vi "Photo_Editor_Project_EE304.vi"() -> ()   [LabVIEW 2019]
panel:
  in  "Save Button":bool
  in  "Blue":i32(slide) scale=0.0..100.0
  in  "Green":i32(slide) scale=0.0..100.0
  in  "Red":i32(slide) scale=0.0..100.0
  in  "Zoom to Fit Canvas":sgl
  out "Image":picture
  in  "Balance Button":bool
  in  "Shadows":i32(slide) scale=0.0..10.0
  in  "Highlights":i32(slide) scale=0.0..10.0
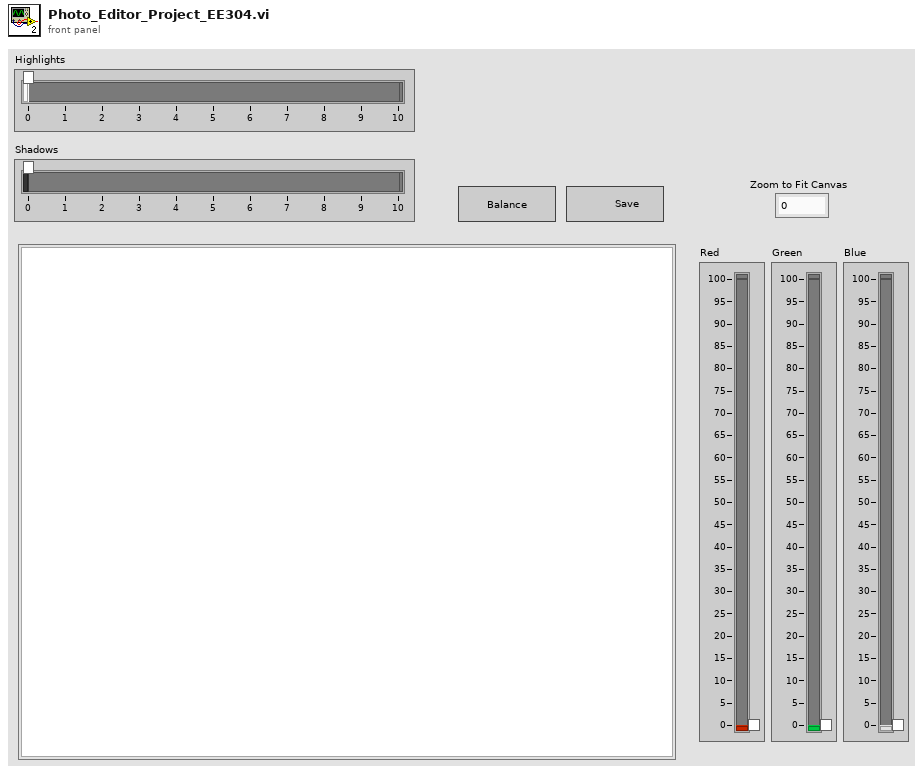
[diagram p1: front panel]
types:
  T1 = typedef "imagedata.ctl" = cluster{"image type":i32, "image depth":i32, "image":u8[], "mask":u8[], "colors":u32[], "Rectangle":cluster{"left":i16, "top":i16, "right":i16, "bottom":i16}}
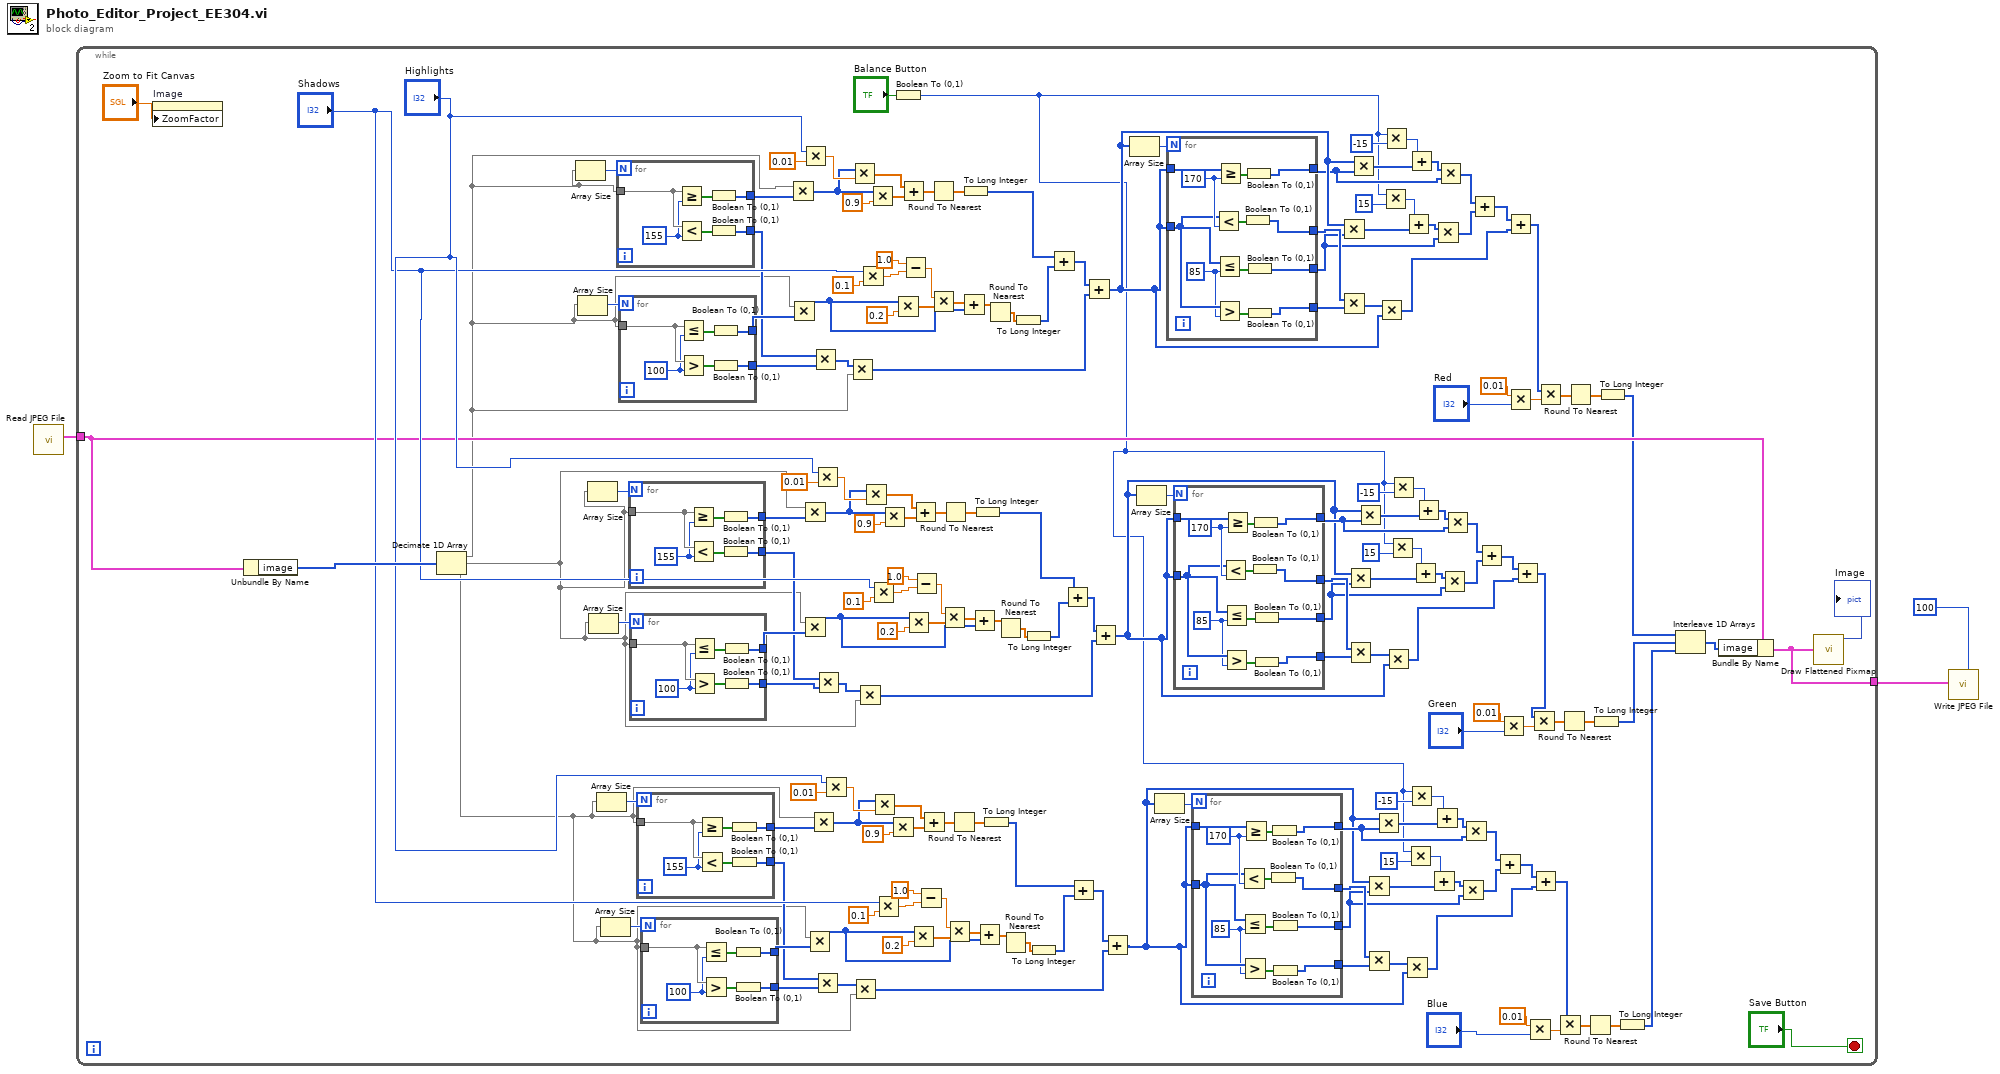
[diagram p0: block diagram]
diagram:
  n1 = call <vilib>:"Read JPEG File.vi"() -> ("image data"=w3:T1)  [unwired: 9 in, 2 out]
  n2 = while {
    tunnel: w3 -> [w90]
    tunnel: [w5] -> w1
    stop <- "Save Button" stop-if-true
    n3 = property on="Image" class="Pict"("ZoomFactor"="Zoom to Fit Canvas") -> ()  [unwired: 2 in, 2 out]
    n4 = Unbundle By Name(w90) -> ("image"=w182:u8[])
    n5 = Decimate 1D Array(w182) -> (w70:u8[], w50:u8[], w29:u8[])
    n6 = Array Size(array=w70) -> (size(s)=w169:i32)
    n7 = Array Size(array=w70) -> (size(s)=w148:i32)
    n8 = Array Size(array=w50) -> (size(s)=w180:i32)
    n9 = Array Size(array=w50) -> (size(s)=w135:i32)
    n10 = Array Size(array=w29) -> (size(s)=w158:i32)
    n11 = Array Size(array=w29) -> (size(s)=w123:i32)
    n12 = for {
      N: w169 -> [_]
      tunnel: w70 -> [w246]
      tunnel: [w247] -> w168
      tunnel: [w243] -> w109
      w245 = u8 155 ("y")
      n13 = Greater Or Equal?(x=w246, y=w245) -> (x >= y?=w248:bool[])
      n14 = Less?(x=w246, y=w245) -> (x < y?=w244:bool[])
      n15 = Boolean To (0,1)(Boolean=w248) -> (0, 1=w247:i16[])
      n16 = Boolean To (0,1)(Boolean=w244) -> (0, 1=w243:i16[])
    }
    n17 = for {
      N: w148 -> [_]
      tunnel: w70 -> [w234]
      tunnel: [w235] -> w146
      tunnel: [w231] -> w108
      w233 = u8 100 ("y")
      n18 = Less Or Equal?(x=w234, y=w233) -> (x <= y?=w236:bool[])
      n19 = Greater?(x=w234, y=w233) -> (0:w232:bool[])
      n20 = Boolean To (0,1)(Boolean=w236) -> (0, 1=w235:i16[])
      n21 = Boolean To (0,1)(Boolean=w232) -> (0, 1=w231:i16[])
    }
    n22 = for {
      N: w180 -> [_]
      tunnel: w50 -> [w252]
      tunnel: [w253] -> w179
      tunnel: [w249] -> w102
      w251 = u8 155 ("y")
      n23 = Greater Or Equal?(x=w252, y=w251) -> (x >= y?=w254:bool[])
      n24 = Less?(x=w252, y=w251) -> (x < y?=w250:bool[])
      n25 = Boolean To (0,1)(Boolean=w254) -> (0, 1=w253:i16[])
      n26 = Boolean To (0,1)(Boolean=w250) -> (0, 1=w249:i16[])
    }
    n27 = for {
      N: w135 -> [_]
      tunnel: w50 -> [w228]
      tunnel: [w229] -> w134
      tunnel: [w225] -> w103
      w227 = u8 100 ("y")
      n28 = Less Or Equal?(x=w228, y=w227) -> (x <= y?=w230:bool[])
      n29 = Greater?(x=w228, y=w227) -> (0:w226:bool[])
      n30 = Boolean To (0,1)(Boolean=w230) -> (0, 1=w229:i16[])
      n31 = Boolean To (0,1)(Boolean=w226) -> (0, 1=w225:i16[])
    }
    n32 = for {
      N: w158 -> [_]
      tunnel: w29 -> [w240]
      tunnel: [w241] -> w157
      tunnel: [w237] -> w98
      w239 = u8 155 ("y")
      n33 = Greater Or Equal?(x=w240, y=w239) -> (x >= y?=w242:bool[])
      n34 = Less?(x=w240, y=w239) -> (x < y?=w238:bool[])
      n35 = Boolean To (0,1)(Boolean=w242) -> (0, 1=w241:i16[])
      n36 = Boolean To (0,1)(Boolean=w238) -> (0, 1=w237:i16[])
    }
    n37 = for {
      N: w123 -> [_]
      tunnel: w29 -> [w222]
      tunnel: [w223] -> w122
      tunnel: [w219] -> w97
      w221 = u8 100 ("y")
      n38 = Less Or Equal?(x=w222, y=w221) -> (x <= y?=w224:bool[])
      n39 = Greater?(x=w222, y=w221) -> (0:w220:bool[])
      n40 = Boolean To (0,1)(Boolean=w224) -> (0, 1=w223:i16[])
      n41 = Boolean To (0,1)(Boolean=w220) -> (0, 1=w219:i16[])
    }
    n42 = Multiply(x=w70, y=w168) -> (x*y=w163:i16[])
    n43 = Multiply(x=w70, y=w146) -> (x*y=w138:i16[])
    n44 = Multiply(x=w50, y=w179) -> (x*y=w174:i16[])
    n45 = Multiply(x=w50, y=w134) -> (x*y=w126:i16[])
    n46 = Multiply(x="Highlights", y=0.01) -> (x*y=w165:dbl)
    n47 = Multiply(x=w29, y=w122) -> (x*y=w114:i16[])
    n48 = Multiply(x=w29, y=w157) -> (x*y=w152:i16[])
    n49 = Multiply(x=w109, y=w108) -> (x*y=w107:i16[])
    n50 = Multiply(x="Highlights", y=0.01) -> (x*y=w176:dbl)
    n51 = Multiply(x=w98, y=w97) -> (x*y=w94:i16[])
    n52 = Multiply(x=w102, y=w103) -> (x*y=w101:i16[])
    n53 = Multiply(x="Highlights", y=0.01) -> (x*y=w154:dbl)
    n54 = Multiply(x=w107, y=w70) -> (x*y=w105:i16[])
    n55 = Multiply(x=w163, y=w165) -> (x*y=w162:dbl[])
    n56 = Multiply(x=w94, y=w29) -> (x*y=w92:i16[])
    n57 = Multiply(x=w101, y=w50) -> (x*y=w99:i16[])
    n58 = Multiply(x="Shadows", y=0.1) -> (x*y=w143:dbl)
    n59 = Multiply(x=w174, y=w176) -> (x*y=w173:dbl[])
    n60 = Multiply(x=w163, y=0.9) -> (x*y=w161:dbl[])
    n61 = Multiply(x="Shadows", y=0.1) -> (x*y=w131:dbl)
    n62 = Multiply(x=w152, y=w154) -> (x*y=w151:dbl[])
    n63 = Multiply(x="Shadows", y=0.1) -> (x*y=w119:dbl)
    n64 = Multiply(x=w174, y=0.9) -> (x*y=w172:dbl[])
    n65 = Multiply(x=w152, y=0.9) -> (x*y=w150:dbl[])
    n66 = Boolean To (0,1)(Boolean="Balance Button") -> (0, 1=w30:i16)
    n67 = Multiply(x=w138, y=0.2) -> (x*y=w140:dbl[])
    n68 = Add(x=w162, y=w161) -> (x+y=w160:dbl[])
    n69 = Subtract(x=1.0, y=w143) -> (x-y=w141:dbl)
    n70 = Multiply(x=w126, y=0.2) -> (x*y=w128:dbl[])
    n71 = Multiply(x=w114, y=0.2) -> (x*y=w116:dbl[])
    n72 = Add(x=w173, y=w172) -> (x+y=w171:dbl[])
    n73 = Subtract(x=1.0, y=w131) -> (x-y=w129:dbl)
    n74 = Subtract(x=1.0, y=w119) -> (x-y=w117:dbl)
    n75 = Add(x=w151, y=w150) -> (x+y=w149:dbl[])
    n76 = Round To Nearest(number=w160) -> (nearest integer value=w167:dbl[])
    n77 = Multiply(x=w141, y=w140) -> (x*y=w139:dbl[])
    n78 = Multiply(x=w129, y=w128) -> (x*y=w127:dbl[])
    n79 = Round To Nearest(number=w171) -> (nearest integer value=w178:dbl[])
    n80 = Multiply(x=w117, y=w116) -> (x*y=w115:dbl[])
    n81 = Round To Nearest(number=w149) -> (nearest integer value=w156:dbl[])
    n82 = Add(x=w139, y=w138) -> (x+y=w137:dbl[])
    n83 = To Long Integer(number=w167) -> (32bit integer=w159:i32[])
    n84 = Add(x=w127, y=w126) -> (x+y=w125:dbl[])
    n85 = To Long Integer(number=w178) -> (32bit integer=w170:i32[])
    n86 = Add(x=w115, y=w114) -> (x+y=w113:dbl[])
    n87 = To Long Integer(number=w156) -> (32bit integer=w95:i32[])
    n88 = Round To Nearest(number=w137) -> (nearest integer value=w136:dbl[])
    n89 = Round To Nearest(number=w125) -> (nearest integer value=w124:dbl[])
    n90 = Round To Nearest(number=w113) -> (nearest integer value=w112:dbl[])
    n91 = To Long Integer(number=w136) -> (32bit integer=w110:i32[])
    n92 = To Long Integer(number=w124) -> (32bit integer=w104:i32[])
    n93 = To Long Integer(number=w112) -> (32bit integer=w96:i32[])
    n94 = Add(x=w159, y=w110) -> (x+y=w106:i32[])
    n95 = Add(x=w170, y=w104) -> (x+y=w100:i32[])
    n96 = Add(x=w95, y=w96) -> (x+y=w93:i32[])
    n97 = Add(x=w106, y=w105) -> (x+y=w85:i32[])
    n98 = Add(x=w100, y=w99) -> (x+y=w51:i32[])
    n99 = Add(x=w93, y=w92) -> (x+y=w31:i32[])
    n100 = Array Size(array=w85) -> (size(s)=w89:i32)
    n101 = Array Size(array=w51) -> (size(s)=w69:i32)
    n102 = Array Size(array=w31) -> (size(s)=w49:i32)
    n103 = for {
      N: w89 -> [_]
      tunnel: w85 -> [w218]
      tunnel: [w216] -> w80
      tunnel: w85 -> [w212]
      tunnel: [w213] -> w88
      tunnel: [w208] -> w75
      tunnel: [w207] -> w87
      w211 = 85 ("y")
      w215 = 170 ("y")
      n104 = Less?(x=w212, y=w215) -> (x < y?=w214:bool[])
      n105 = Less Or Equal?(x=w212, y=w211) -> (x <= y?=w210:bool[])
      n106 = Greater?(x=w212, y=w211) -> (0:w209:bool[])
      n107 = Greater Or Equal?(x=w218, y=w215) -> (x >= y?=w217:bool[])
      n108 = Boolean To (0,1)(Boolean=w214) -> (0, 1=w213:i16[])
      n109 = Boolean To (0,1)(Boolean=w217) -> (0, 1=w216:i16[])
      n110 = Boolean To (0,1)(Boolean=w210) -> (0, 1=w208:i16[])
      n111 = Boolean To (0,1)(Boolean=w209) -> (0, 1=w207:i16[])
    }
    n112 = for {
      N: w69 -> [_]
      tunnel: w51 -> [w206]
      tunnel: [w204] -> w61
      tunnel: w51 -> [w200]
      tunnel: [w201] -> w68
      tunnel: [w196] -> w56
      tunnel: [w195] -> w67
      w199 = 85 ("y")
      w203 = 170 ("y")
      n113 = Less?(x=w200, y=w203) -> (x < y?=w202:bool[])
      n114 = Less Or Equal?(x=w200, y=w199) -> (x <= y?=w198:bool[])
      n115 = Greater?(x=w200, y=w199) -> (0:w197:bool[])
      n116 = Greater Or Equal?(x=w206, y=w203) -> (x >= y?=w205:bool[])
      n117 = Boolean To (0,1)(Boolean=w202) -> (0, 1=w201:i16[])
      n118 = Boolean To (0,1)(Boolean=w205) -> (0, 1=w204:i16[])
      n119 = Boolean To (0,1)(Boolean=w198) -> (0, 1=w196:i16[])
      n120 = Boolean To (0,1)(Boolean=w197) -> (0, 1=w195:i16[])
    }
    n121 = for {
      N: w49 -> [_]
      tunnel: w31 -> [w194]
      tunnel: [w192] -> w41
      tunnel: w31 -> [w188]
      tunnel: [w189] -> w48
      tunnel: [w184] -> w36
      tunnel: [w183] -> w47
      w187 = 85 ("y")
      w191 = 170 ("y")
      n122 = Less?(x=w188, y=w191) -> (x < y?=w190:bool[])
      n123 = Less Or Equal?(x=w188, y=w187) -> (x <= y?=w186:bool[])
      n124 = Greater?(x=w188, y=w187) -> (0:w185:bool[])
      n125 = Greater Or Equal?(x=w194, y=w191) -> (x >= y?=w193:bool[])
      n126 = Boolean To (0,1)(Boolean=w190) -> (0, 1=w189:i16[])
      n127 = Boolean To (0,1)(Boolean=w193) -> (0, 1=w192:i16[])
      n128 = Boolean To (0,1)(Boolean=w186) -> (0, 1=w184:i16[])
      n129 = Boolean To (0,1)(Boolean=w185) -> (0, 1=w183:i16[])
    }
    n130 = Multiply(x=w85, y=w75) -> (x*y=w77:i32[])
    n131 = Multiply(x=w88, y=w87) -> (x*y=w86:i16[])
    n132 = Multiply(x=w51, y=w56) -> (x*y=w58:i32[])
    n133 = Multiply(x=w68, y=w67) -> (x*y=w66:i16[])
    n134 = Multiply(x=w85, y=w80) -> (x*y=w82:i32[])
    n135 = Multiply(x=w51, y=w61) -> (x*y=w63:i32[])
    n136 = Multiply(x=w31, y=w36) -> (x*y=w38:i32[])
    n137 = Multiply(x=w48, y=w47) -> (x*y=w46:i16[])
    n138 = Multiply(x=w31, y=w41) -> (x*y=w43:i32[])
    n139 = Multiply(x=w86, y=w85) -> (x*y=w71:i32[])
    n140 = Multiply(x=w30, y=i16 15) -> (x*y=w78:i16)
    n141 = Multiply(x=w30, y=-15) -> (x*y=w83:i32)
    n142 = Multiply(x=w66, y=w51) -> (x*y=w52:i32[])
    n143 = Multiply(x=w30, y=i16 15) -> (x*y=w59:i16)
    n144 = Multiply(x=w30, y=-15) -> (x*y=w64:i32)
    n145 = Multiply(x=w46, y=w31) -> (x*y=w32:i32[])
    n146 = Add(x=w78, y=w77) -> (x+y=w76:i32[])
    n147 = Multiply(x=w30, y=i16 15) -> (x*y=w39:i16)
    n148 = Add(x=w83, y=w82) -> (x+y=w81:i32[])
    n149 = Multiply(x=w30, y=-15) -> (x*y=w44:i32)
    n150 = Add(x=w59, y=w58) -> (x+y=w57:i32[])
    n151 = Add(x=w64, y=w63) -> (x+y=w62:i32[])
    n152 = Add(x=w39, y=w38) -> (x+y=w37:i32[])
    n153 = Add(x=w44, y=w43) -> (x+y=w42:i32[])
    n154 = Multiply(x=w76, y=w75) -> (x*y=w73:i32[])
    n155 = Multiply(x=w81, y=w80) -> (x*y=w74:i32[])
    n156 = Multiply(x=w57, y=w56) -> (x*y=w54:i32[])
    n157 = Multiply(x=w62, y=w61) -> (x*y=w55:i32[])
    n158 = Multiply(x=w37, y=w36) -> (x*y=w34:i32[])
    n159 = Multiply(x=w42, y=w41) -> (x*y=w35:i32[])
    n160 = Add(x=w74, y=w73) -> (x+y=w72:i32[])
    n161 = Add(x=w55, y=w54) -> (x+y=w53:i32[])
    n162 = Add(x=w35, y=w34) -> (x+y=w33:i32[])
    n163 = Multiply(x=0.01, y="Green") -> (x*y=w21:dbl)
    n164 = Add(x=w72, y=w71) -> (x+y=w25:i32[])
    n165 = Multiply(x=0.01, y="Red") -> (x*y=w26:dbl)
    n166 = Add(x=w53, y=w52) -> (x+y=w17:i32[])
    n167 = Multiply(x=0.01, y="Blue") -> (x*y=w15:dbl)
    n168 = Multiply(x=w17, y=w21) -> (x*y=w20:dbl[])
    n169 = Add(x=w33, y=w32) -> (x+y=w11:i32[])
    n170 = Multiply(x=w25, y=w26) -> (x*y=w24:dbl[])
    n171 = Multiply(x=w11, y=w15) -> (x*y=w14:dbl[])
    n172 = Round To Nearest(number=w20) -> (nearest integer value=w19:dbl[])
    n173 = Round To Nearest(number=w24) -> (nearest integer value=w23:dbl[])
    n174 = Round To Nearest(number=w14) -> (nearest integer value=w13:dbl[])
    n175 = To Long Integer(number=w19) -> (32bit integer=w6:i32[])
    n176 = To Long Integer(number=w23) -> (32bit integer=w8:i32[])
    n177 = To Long Integer(number=w13) -> (32bit integer=w7:i32[])
    n178 = Interleave 1D Arrays(w8, w6, w7) -> (w9:i32[])
    n179 = Bundle By Name(cluster=w90, "image"=w9) -> (w5:T1)
    n180 = call <vilib>:"Draw Flattened Pixmap.vi"("image data"=w5) -> ("new picture"=→"Image":picture)  [unwired: 8 in]
  }
  n181 = call <vilib>:"Write JPEG File.vi"("quality (80)"=100, "image data"=w1) -> ()  [unwired: 8 in, 2 out]
